vi "Request Task Setpoint.vi"(7 "Task Ident":string, 8 "error in":errorcluster, 10 "Setpoint Ident":string, 11 "Series Actor in":refnum<class "Series Actor.lvclass">) -> (0 "error out":errorcluster, 3 "Series Actor out":refnum<class "Series Actor.lvclass">)   [LabVIEW 2024, in "Series Actor.lvlib" / "Series Actor.lvclass"]
uses:
  Series Actor.lvclass
  Series Actor.lvclass/Series Actor.ctl
  Task/ITask Actor/ITask Actor Messages/Publish Setpoint Msg/Publish Setpoint Msg.lvclass
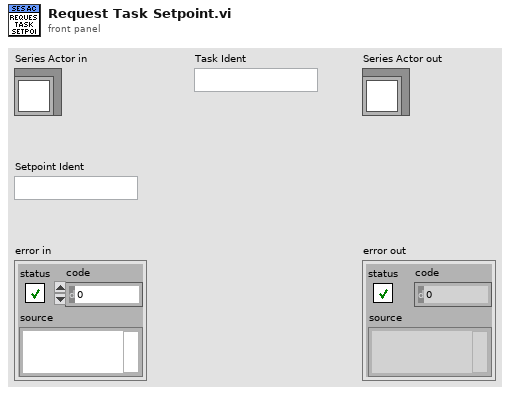
[diagram p1: front panel]
types:
  T1 = map{string, refnum<class "Message Enqueuer.lvclass">}
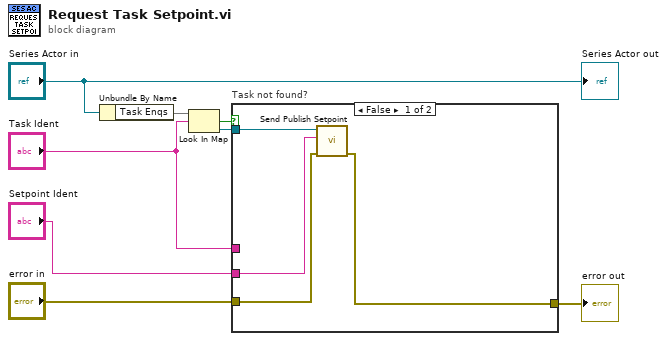
[diagram p0: block diagram]
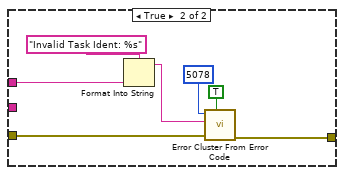
[diagram p2: hidden frame]
diagram:
  n1 = Unbundle By Name("Series Actor in") -> ("Task Enqs"=w7:T1)
  n2 = Look In Map(map=w7, key="Task Ident") -> (key not found?=w6:bool, value=w5:refnum<class "Message Enqueuer.lvclass">)  [unwired: 1 in]
  n3 = case "Task not found?" shown="False" w6 {
    tunnel: w5 -> [w12 _]
    tunnel: "error in" -> [w11 w19]
    tunnel: [w9 w18] -> w3
    tunnel: "Task Ident" -> [_ w13]
    tunnel: "Setpoint Ident" -> [w10 _]
    frame False {
      n4 = call "Send Publish Setpoint.vi"("error in (no error)"=w11, "Ident"=w10, "Message Enqueuer"=w12) -> ("error out"=w9:errorcluster)  [unwired: 7 in, 1 out]
    }
    frame True {
      n5 = Format Into String(format string="Invalid Task Ident: %s", w13) -> (resulting string=w14:string)  [unwired: 2 in, 1 out]
      n6 = call <vilib>:"Error Cluster From Error Code.vi"("show call chain? (False)"=TRUE, "error in (no error)"=w19, "error message (\"\")"=w14, "error code (0)"=5078) -> ("error out"=w18:errorcluster)  [unwired: 5 in]
    }
  }
  "error out" <- w3
  "Series Actor out" <- "Series Actor in"
